vi "Handle Error.vi"(8 "error in (no error)":errorcluster, 11 "InferenceTCP in":refnum<class "InferenceTCP.lvclass">) -> (0 "error out":errorcluster, 2 "stop actor?":bool=TRUE, 3 "InferenceTCP out":refnum<class "InferenceTCP.lvclass">)   [LabVIEW 2019, in "InferenceTCP.lvlib" / "InferenceTCP.lvclass"]
doc: "(<B>Filename</B>: Actor Framework.lvlib:Actor.lvclass:Handle Error.vi)\n\nDefines how the actor handles an error that occurred while processing a message. By default, this method does nothing except stop the actor."
uses:
  InferenceTCP.lvclass
  C:/Program Files/National Instruments/LabVIEW 2019/vi.lib/ActorFramework/Actor/Actor.lvclass
  <vilib>/ActorFramework/Actor/Actor.lvclass/Actor.ctl
  <vilib>/ActorFramework/Message Enqueuer/Message Enqueuer.lvclass/Message Enqueuer.ctl
  InferenceTCP.lvclass/InferenceTCP.ctl
  <vilib>/ActorFramework/Message Enqueuer/Init from Existing Queue.vi
  <vilib>/ActorFramework/Message Enqueuer/Enqueue.vi
  InferenceTCP Messages/Connect Msg/Connect Msg.lvclass
  C:/Program Files/National Instruments/LabVIEW 2019/vi.lib/ActorFramework/Message/Message.lvclass
  <vilib>/ActorFramework/Message Priority Queue/Priority Enqueue.vi
  <vilib>/ActorFramework/Message Enqueuer/Message Enqueuer.lvclass
  Inference/Inference/Inference.lvclass
  <vilib>/ActorFramework/Actor/Actor.lvclass
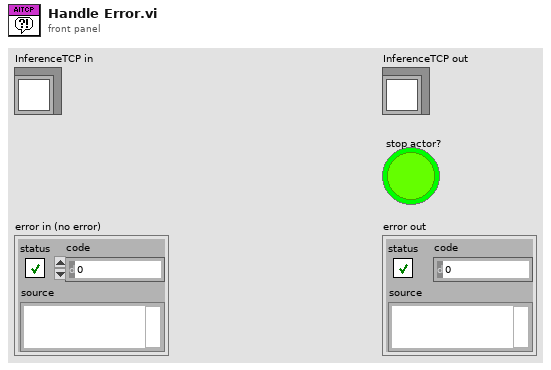
[diagram p1: front panel]
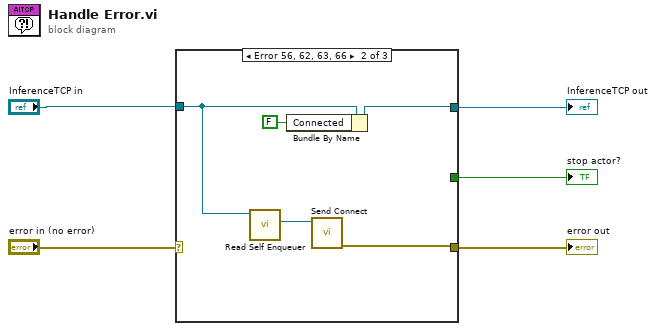
[diagram p0: block diagram]
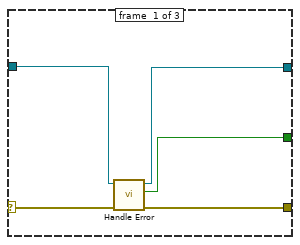
[diagram p2: hidden frame]
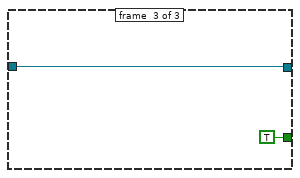
[diagram p3: hidden frame]
diagram:
  n1 = case shown="Error 56, 62, 63, 66" "error in (no error)" {
    selector: "error in (no error)" -> [w7 _ _]
    tunnel: [w10 w14 _] -> w1
    tunnel: [w9 _ TRUE ("stop actor?")] -> w2
    tunnel: [w8 w12 w17] -> w3
    tunnel: "InferenceTCP in" -> [w6 w13 w17]
    frame #0 {
      n2 = call-parent "Handle Error.vi"("error in (no error)"=w7, "Actor in"=w6) -> ("error out"=w10:errorcluster, "stop actor?"=w9:bool, "Actor out"=w8:refnum<class "InferenceTCP.lvclass">)  [unwired: 7 in]
    }
    frame #1 {
      n3 = call <vilib>:"Read Self Enqueuer.vi"("Actor"=w13) -> ("Self Enqueuer"=w15:refnum<class "Message Enqueuer.lvclass">)  [unwired: 10 in]
      n4 = Bundle By Name(cluster=w13, "Connected"=FALSE) -> (w12:refnum<class "InferenceTCP.lvclass">)
      n5 = call "Send Connect.vi"("Message Enqueuer"=w15) -> ("error out"=w14:errorcluster)  [unwired: 9 in, 1 out]
    }
    frame #2 {
    }
  }
  "InferenceTCP out" <- w3
  "error out" <- w1
  "stop actor?" <- w2
